vi "Get Version.vi"(8 "error in (no error)":errorcluster, 10 "Number of Digits for Version(4)":i32=4, 11 "File Path (Optional)":path) -> (0 "error out":errorcluster, 3 "Version":string)   [LabVIEW 2016, in "SLL Application.lvlib"]
doc: "Returns the version for the file path specified. \n\nIf the file path is empty, it would get the version of the current application."
uses:
  SLL Application.lvlib
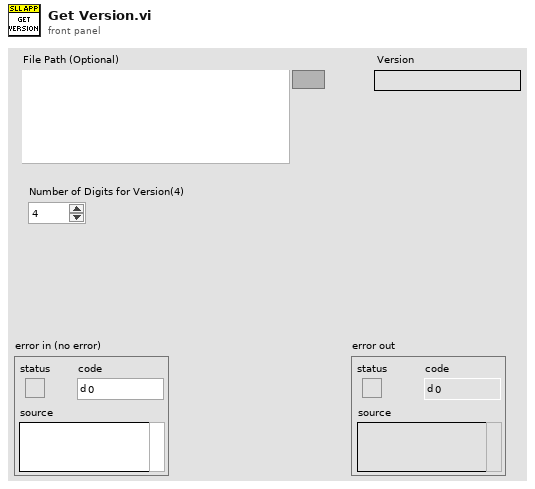
[diagram p1: front panel]
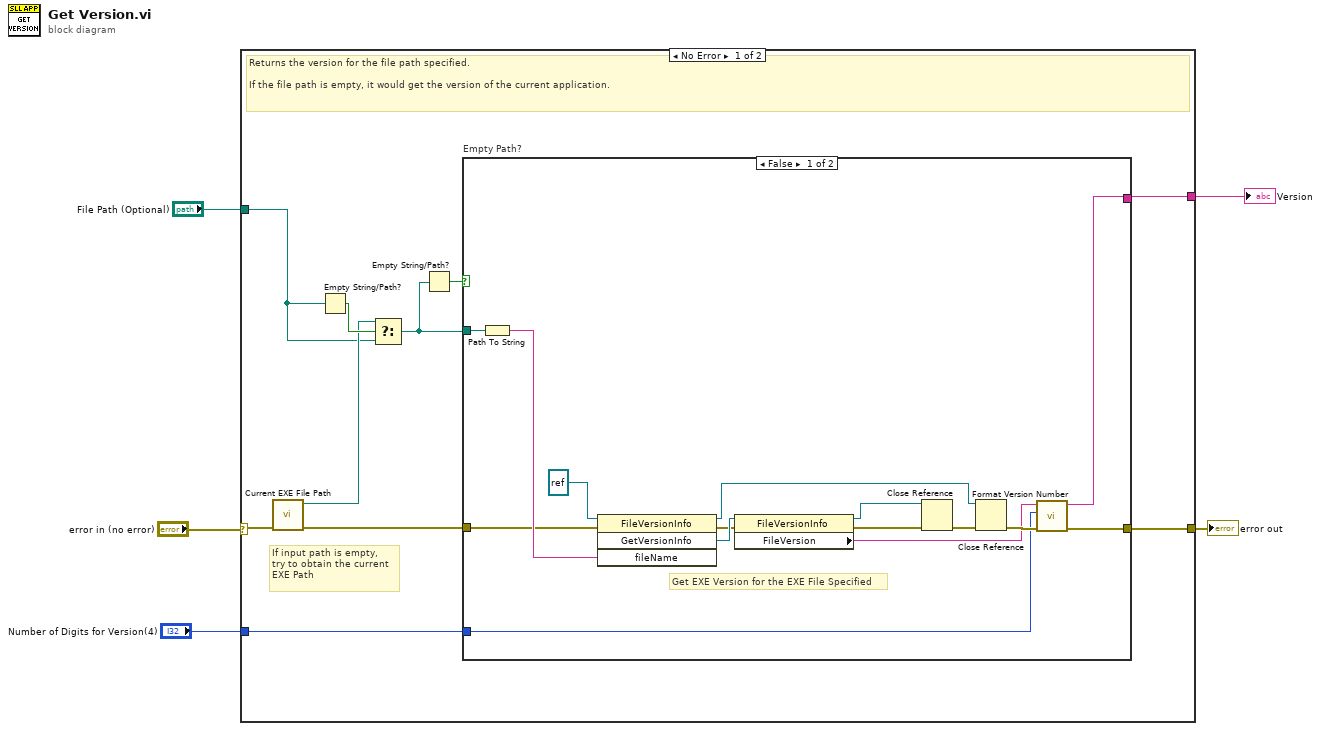
[diagram p0: block diagram]
diagram:
  n1 = case shown="No Error" "error in (no error)" {
    selector: "error in (no error)" -> [w12 w32]
    tunnel: "File Path (Optional)" -> [w8 _]
    tunnel: [w15 w32] -> w3
    tunnel: [w14 _] -> w2
    tunnel: "Number of Digits for Version(4)" -> [w13 _]
    frame No Error {
      # "If input path is empty,\ntry to obtain the current\nEXE Path"
      # "Returns the version for the file path specified. \n\nIf the file path is empty, it would get the version of the current application."
      n2 = call "Current EXE File Path.vi"("error in (no error)"=w12) -> ("error out"=w11:errorcluster, "Current EXE Path"=w9:path)  [unwired: 9 in]
      n3 = Empty String/Path?(string/path=w8) -> (empty?=w10:bool)
      n4 = Select(t=w9, s=w10, f=w8) -> (s? t:f=w6:path)
      n5 = Empty String/Path?(string/path=w6) -> (empty?=w7:bool)
      n6 = case "Empty Path?" shown="False" w7 {
        tunnel: [w21 w31] -> w15
        tunnel: [w19 _] -> w14
        tunnel: w13 -> [w18 _]
        tunnel: w11 -> [w17 w31]
        tunnel: w6 -> [w16 _]
        frame False {
          # "Get EXE Version for the EXE File Specified"
          n7 = Path To String(path=w16) -> (string=w29:string)
          n8 = invoke on="Invoke Node" class="FileVersionInfo" method="GetVersionInfo"(reference=refnum<k24> refnum, error in=w17, "fileName"=w29) -> (reference out=w23:refnum<k24>, error out=w27:errorcluster, "GetVersionInfo"=w28:refnum<k24>)  [unwired: 1 in, 1 out]
          n9 = property on="Property Node" class="FileVersionInfo"(reference=w28, error in=w27) -> (reference out=w26:refnum<k24>, error out=w25:errorcluster, "FileVersion"=w20:string)
          n10 = Close Reference(reference=w26, error in (no error)=w25) -> (error out=w24:errorcluster)
          n11 = Close Reference(reference=w23, error in (no error)=w24) -> (error out=w22:errorcluster)
          n12 = call "Format Version Number.vi"("error in (no error)"=w22, "Number of Digits (4)"=w18, "Version In"=w20) -> ("error out"=w21:errorcluster, "Version Out"=w19:string)  [unwired: 7 in]
        }
        frame True {
          # "Empty Path. Ignore."
        }
      }
    }
    frame Error {
    }
  }
  "error out" <- w3
  "Version" <- w2
